vi "Autonomous Independent.vi"() -> ()   [LabVIEW 2016]
doc: "This VI is called when autonomous begins, and will automatically be terminated when autonomous ends. You can carry out timed or sensor driven robot movement independently without needing to return to the caller."
uses:
  Robot Global Data.vi
  <vilib>/addons/control/pid/pid.llb/PID (DBL).vi
  navX Library v2/navX Library v2.lvlib
  <vilib>/addons/control/pid/NI_PID_pid.lvlib
  <vilib>/Rock Robotics/Network Tables/NT Read String.vi
panel:
  out "x+y":dbl
  out "x-y":dbl
  out "Numeric 2":i32
  out "elapsed time":i32
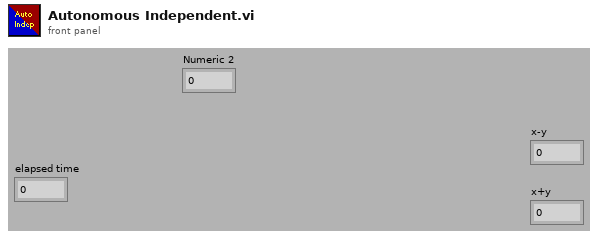
[diagram p1: front panel]
types:
  T1 = typedef "navX Library v2.lvlib/Z900_navX_DeviceTypeDef.ctl" = cluster{"Interface":cluster{"Protocol":T2, "Update Rate (4Hz-100Hz)":u8, "navX Open TypeDef":variant}, "Notify Packet":refnum<notifier>, "Loop VI Refnum":refnum<vi>, "Ready to Close Occurrence Refnum":refnum<k4>}
  T2 = typedef "navX Library v2.lvlib/Z900_navX_ProtocolTypeDef.ctl" = enum16{"SERIAL", "I2C", "SPI"}
  T3 = typedef "WPI_EncoderDevRef.ctl" = cluster{"DevStatus":errorcluster, "EncoderIndex":T4, "CounterIndex":T5, "DistancePerCount":dbl, "Decoding Type":T6}
  T4 = typedef "FPGA_EncoderIdx.ctl" = enum8{"Enc 0", "Enc 1", "Enc 2", "Enc 3", "Enc 4", "Enc 5", "Enc 6", "Enc 7", "Invalid"}
  T5 = typedef "FPGA_CounterCtrSystemIndex.ctl" = enum8{"Ctr 0", "Ctr 1", "Ctr 2", "Ctr 3", "Ctr 4", "Ctr 5", "Ctr 6", "Ctr 7", "Invalid"}
  T6 = typedef "WPI_EncoderType.ctl" = enum16{"1x", "2x", "4x"}
  T7 = cluster{"proportional gain (Kc)":dbl, "integral time (Ti, min)":dbl, "derivative time (Td, min)":dbl}
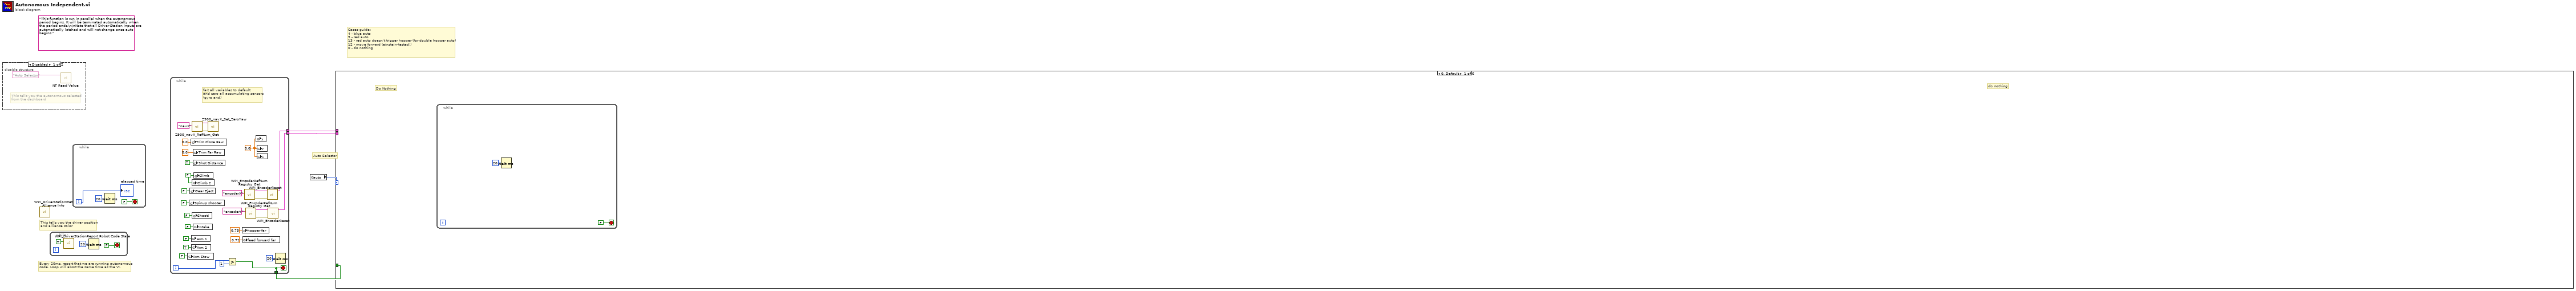
[diagram p0: block diagram]
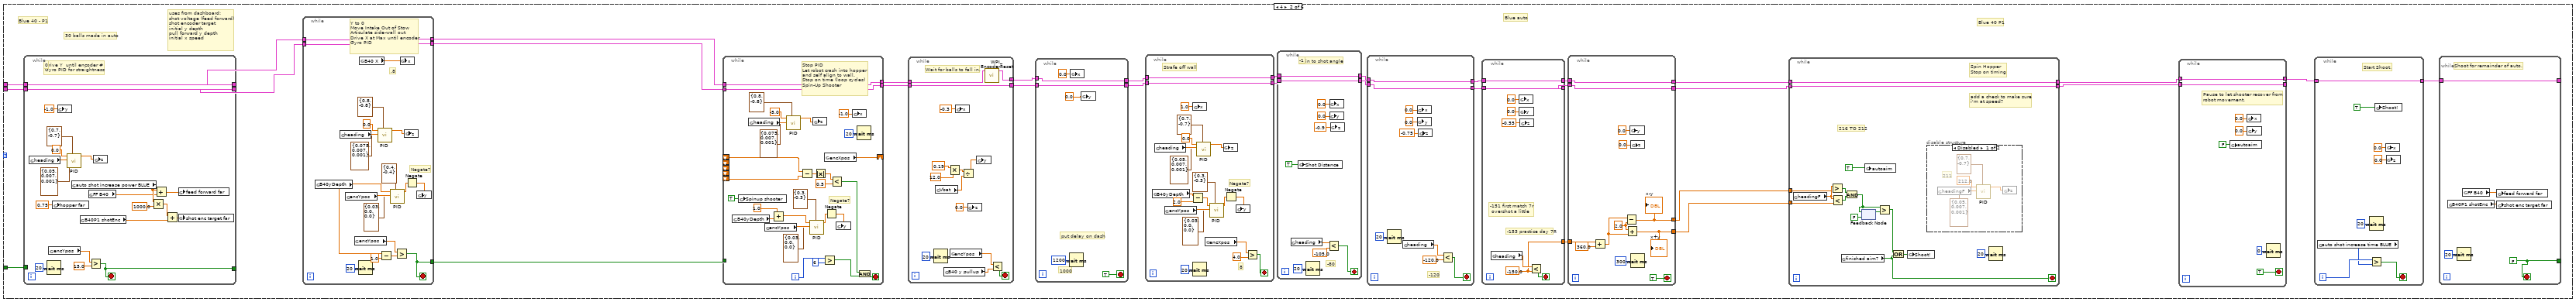
[diagram p2: hidden frame]
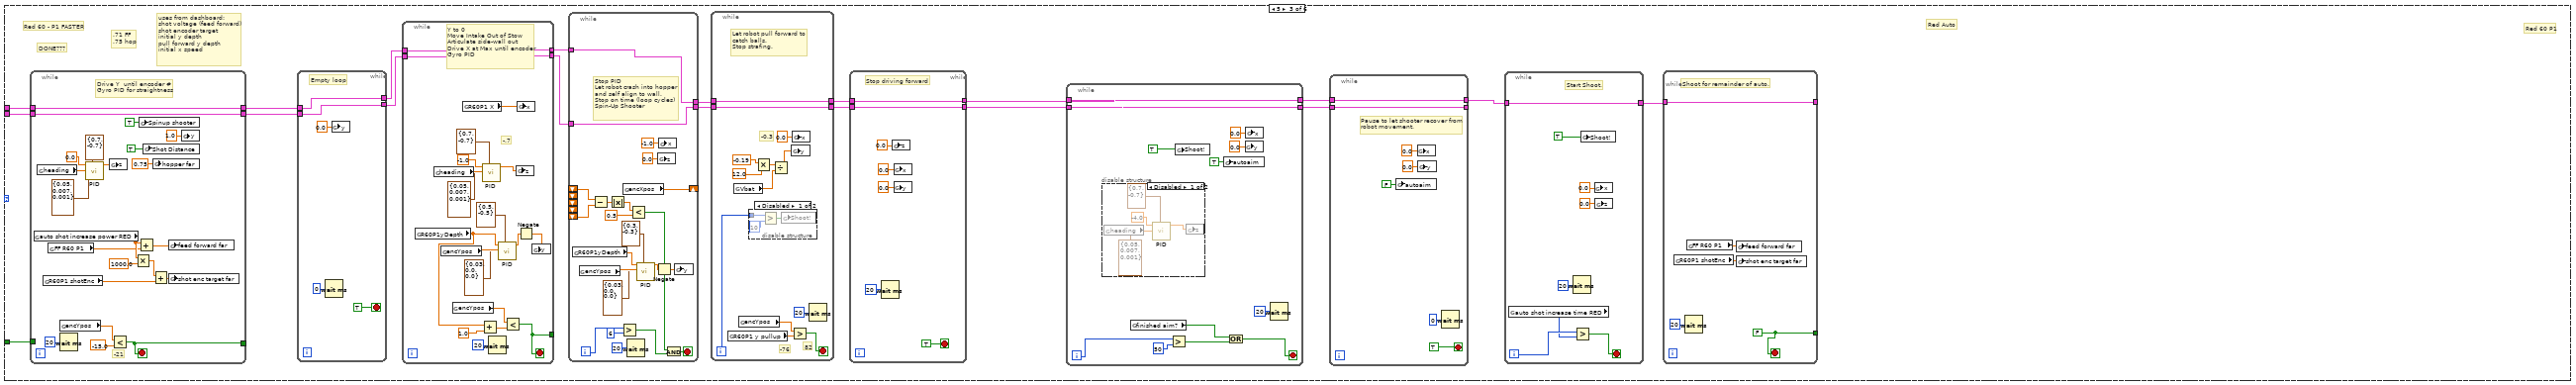
[diagram p4: hidden frame]
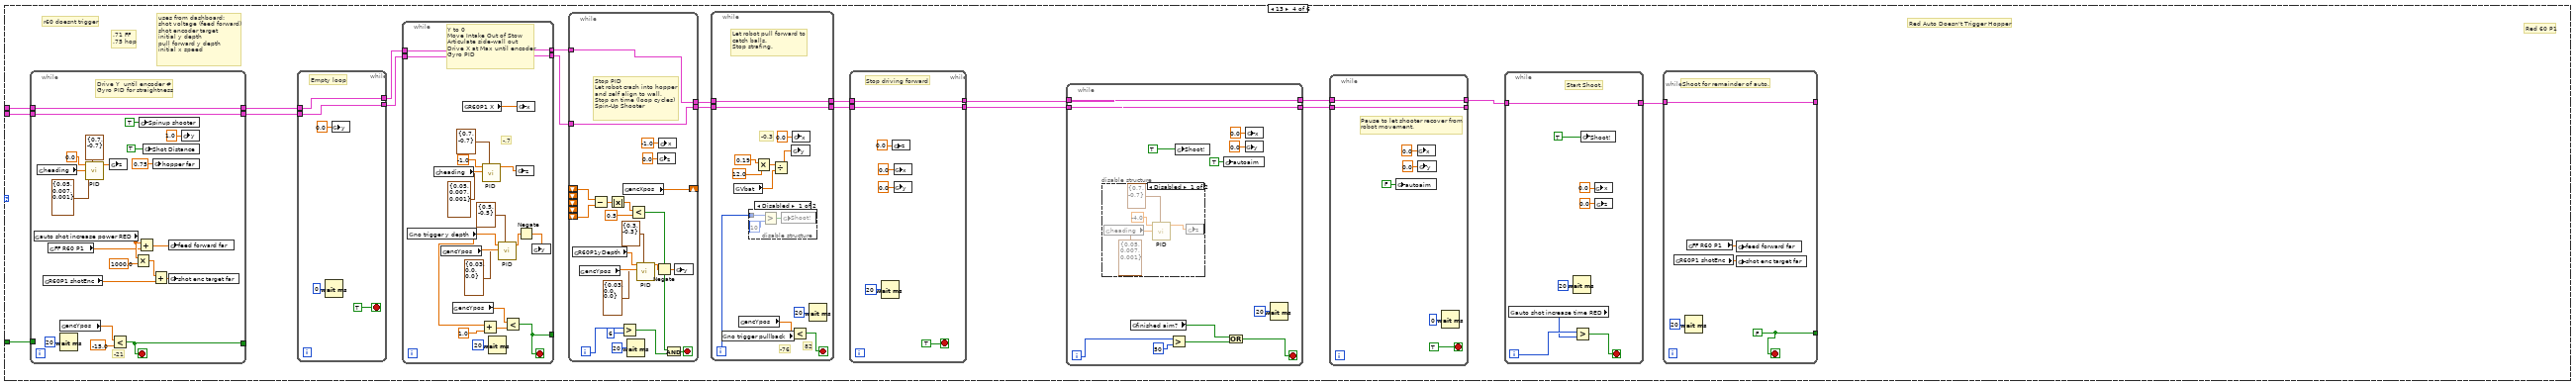
[diagram p7: hidden frame]
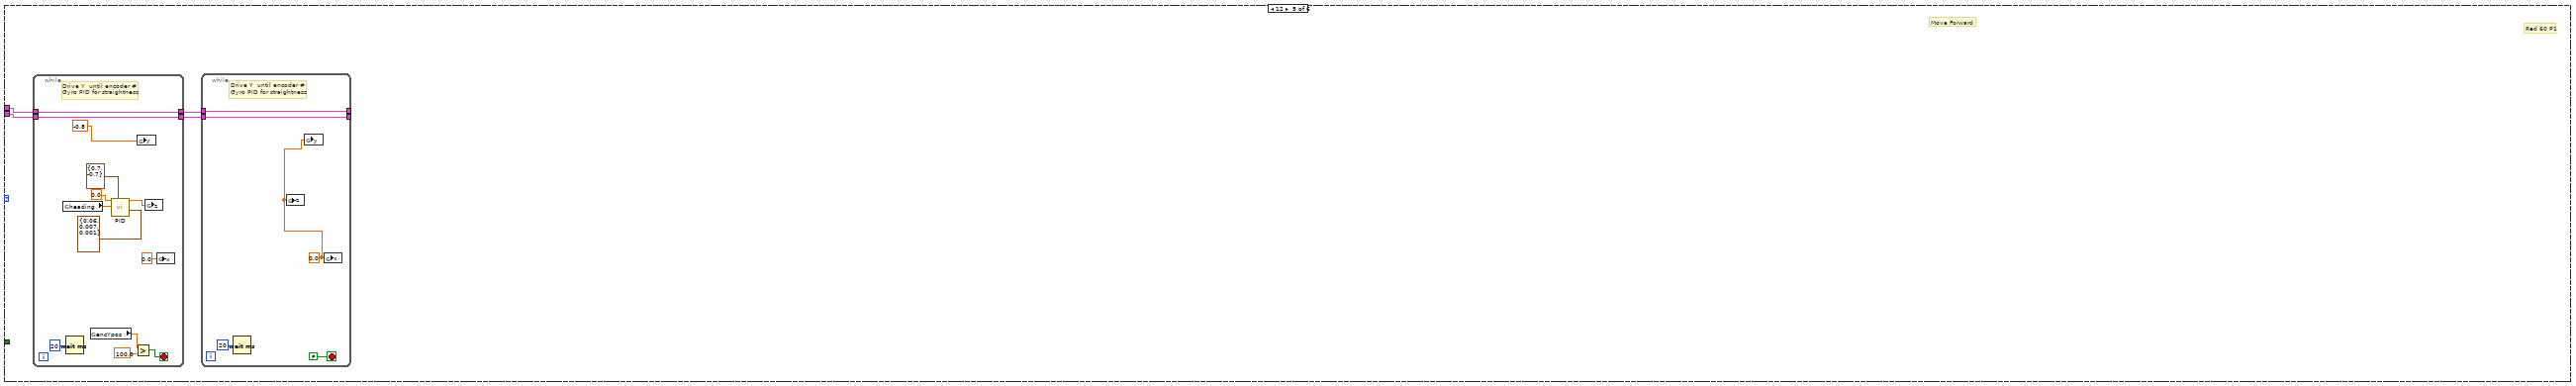
[diagram p10: hidden frame]
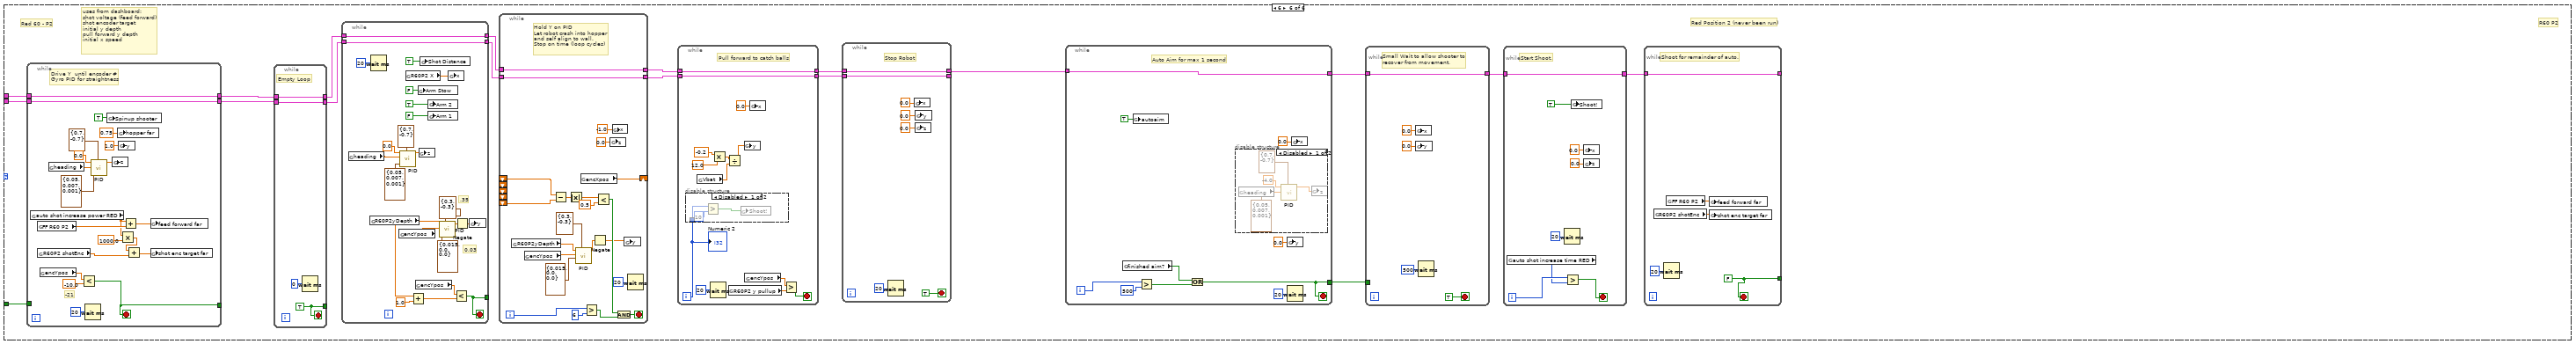
[diagram p11: hidden frame]
diagram:
  (unwired) "This function is run in parallel when the autonomous period begins. It will be terminated automatically when the period ends.\n\nNote that all Driver Station inputs are automatically latched and will not change once auto begins."
  # "Cases guide:\n4 - blue auto\n5 - red auto\n13 - red auto doesn't trigger hopper (for double hopper auto)\n12 - move forward (einstein-tested!)\n0 - do nothing"
  # "Auto Selector"
  # "Every 20ms, report that we are running autonomous\ncode. Loop will abort the same time as the VI."
  # "This tells you the driver position\nand alliance color"
  n1 = disable-structure shown="Disabled" {
    frame Disabled {
      # "This tells you the autonomous selected\nfrom the dashboard"
      n2 = call-poly <vilib>:"NT Read Value.vi"("Name"="Auto Selector") -> ()  [unwired: 9 in, 2 out]
    }
    frame Enabled {
    }
  }
  n3 = call <vilib>:"WPI_DriverStationGet Alliance Info.vi"() -> ()  [unwired: 12 out]
  n4 = while {
    stop <- FALSE stop-if-true
    n5 = call <vilib>:"WPI_DriverStationReport Robot Code State.vi"("Autonomous"=TRUE) -> ()  [unwired: 10 in, 1 out]
    n6 = Wait (ms)(milliseconds to wait=u32 20) -> ()  [unwired: 1 out]
  }
  n7 = while {
    i -> [w9]
    stop <- FALSE stop-if-true
    n8 = Wait (ms)(milliseconds to wait=u32 20) -> ()  [unwired: 1 out]
    "elapsed time" <- w9
  }
  n9 = while {
    tunnel: [w18] -> w4
    tunnel: [w21] -> w2
    tunnel: [w12] -> w1
    i -> [w20]
    stop <- w18 stop-if-true
    w28 = 0.0 ("y")
    w36 = FALSE ("Climb")
    # "far"
    # "Set all variables to default\nand zero all accumulating sensors\n(gyro and)"
    n10 = global write "Robot Global Data.vi" "Arm Stow"(FALSE ("Arm Stow")) -> ()
    n11 = global write "Robot Global Data.vi" "Spinup shooter"(FALSE ("Spinup shooter")) -> ()
    n12 = global write "Robot Global Data.vi" "Gear Eject"(FALSE ("Gear Eject")) -> ()
    n13 = global write "Robot Global Data.vi" "Trim Close Raw"(0.0 ("Trim Close Raw")) -> ()
    n14 = global write "Robot Global Data.vi" "Arm 1"(FALSE ("Arm 1")) -> ()
    n15 = global write "Robot Global Data.vi" "Arm 2"(TRUE ("Arm 2")) -> ()
    n16 = call "Z900_navX_RefNum_Get.vi"("refnum name"="navX") -> ("error out"=w15:errorcluster, "navX Device"=w14:T1)  [unwired: 9 in]
    n17 = global write "Robot Global Data.vi" "Climb 2"(w36) -> ()
    n18 = global write "Robot Global Data.vi" "Shoot!"(FALSE ("Shoot!")) -> ()
    n19 = global write "Robot Global Data.vi" "Trim Far Raw"(0.0 ("Trim Close Raw")) -> ()
    n20 = global write "Robot Global Data.vi" "Shot Distance"(TRUE ("Shot Distance")) -> ()
    n21 = global write "Robot Global Data.vi" "Intake"(FALSE ("Intake")) -> ()
    n22 = global write "Robot Global Data.vi" "Climb"(w36) -> ()
    n23 = call "Z900_navX_Set_ZeroYaw.vi"("error in (no error)"=w15, "navX Device"=w14) -> ()  [unwired: 8 in, 2 out]
    n24 = Greater?(x=w20, y=1) -> (0:w18:bool)
    n25 = global write "Robot Global Data.vi" "hopper far"(0.75 ("hopper far")) -> ()
    n26 = global write "Robot Global Data.vi" "feed forward far"(0.71 ("feed forward far")) -> ()
    n27 = call <vilib>:"WPI_EncoderRefNum Registry Get.vi"("refnum name"="encoderX") -> ("error out"=w26:errorcluster, "EncoderDevRef"=w27:T3)  [unwired: 9 in]
    n28 = call <vilib>:"WPI_EncoderRefNum Registry Get.vi"("refnum name"="encoderY") -> ("error out"=w24:errorcluster, "EncoderDevRef"=w25:T3)  [unwired: 9 in]
    n29 = global write "Robot Global Data.vi" "x"(w28) -> ()
    n30 = global write "Robot Global Data.vi" "y"(w28) -> ()
    n31 = global write "Robot Global Data.vi" "z"(w28) -> ()
    n32 = call <vilib>:"WPI_EncoderReset.vi"("error in (no error)"=w26, "EncoderDevRef"=w27) -> ("EncoderDevRef"=w21:T3)  [unwired: 8 in, 1 out]
    n33 = call <vilib>:"WPI_EncoderReset.vi"("error in (no error)"=w24, "EncoderDevRef"=w25) -> ("EncoderDevRef"=w12:T3)  [unwired: 8 in, 1 out]
    n34 = Wait (ms)(milliseconds to wait=u32 20) -> ()  [unwired: 1 out]
  }
  n35 = global read "Robot Global Data.vi" "auto"() -> (w3:i32)
  n36 = case shown="0, Default" w3 {
    tunnel: w4 -> [_ w73 w279 w426 _ w594]
    tunnel: w2 -> [_ w72 w278 w425 w558 w593]
    tunnel: w1 -> [_ w71 w277 w424 w557 w592]
    frame 0, Default {
      # "Do Nothing"
      # "do nothing"
      n37 = while {
        stop <- FALSE stop-if-true
        n38 = Wait (ms)(milliseconds to wait=u32 20) -> ()  [unwired: 1 out]
      }
    }
    frame 4 {
      # "Blue auto"
      # "uses from dashboard:\nshot voltage (feed forward)\nshot encoder target\ninitial y depth\npull forward y depth\ninitial x speed"
      # "30 balls made in auto"
      # "Blue 40 P1"
      # "Blue 40 - P1"
      n39 = while {
        tunnel: w73 -> [_]
        tunnel: [w252] -> _
        tunnel: [w251] -> w67
        tunnel: w72 -> [w251]
        tunnel: [w250] -> w66
        tunnel: w71 -> [w250]
        stop <- w252 stop-if-true
        # "0"
        # "Drive Y  until encoder #\nGyro PID for straightness"
        n40 = global read "Robot Global Data.vi" "heading"() -> (w258:dbl)
        n41 = Wait (ms)(milliseconds to wait=u32 20) -> ()  [unwired: 1 out]
        n42 = global read "Robot Global Data.vi" "encYpos"() -> (w255:dbl)
        n43 = global write "Robot Global Data.vi" "hopper far"(0.75 ("hopper far")) -> ()
        n44 = global write "Robot Global Data.vi" "y"(-1.0 ("y")) -> ()
        n45 = call-poly <vilib>:"PID.vi"("output range"=cluster{"output high":dbl, "output low":dbl} {"output high"=0.7, "output low"=-0.7}, "PID gains"=T7 {"proportional gain (Kc)"=0.05, "integral time (Ti, min)"=0.007, "derivative time (Td, min)"=0.001}, "process variable"=w258, "setpoint"=0.0) -> ("output"=w256:dbl)  [unwired: 6 in, 1 out]
        n46 = global read "Robot Global Data.vi" "auto shot increase power BLUE"() -> (w246:dbl)
        n47 = global read "Robot Global Data.vi" "B40P1 shotEnc"() -> (w243:dbl)
        n48 = global read "Robot Global Data.vi" "FF B40"() -> (w242:dbl)
        n49 = Greater?(x=w255, y=15.0) -> (0:w252:bool)
        n50 = global write "Robot Global Data.vi" "z"(w256) -> ()
        n51 = Multiply(x=w246, y=1000.0) -> (x*y=w244:dbl)
        n52 = Add(x=w246, y=w242) -> (x+y=w247:dbl)
        n53 = Add(x=w244, y=w243) -> (x+y=w241:dbl)
        n54 = global write "Robot Global Data.vi" "feed forward far"(w247) -> ()
        n55 = global write "Robot Global Data.vi" "shot enc target far"(w241) -> ()
      }
      n56 = while {
        tunnel: [w240] -> w70
        tunnel: w67 -> [w240]
        tunnel: w66 -> [w239]
        tunnel: [w239] -> w69
        tunnel: [w232] -> w68
        stop <- w232 stop-if-true
        # ".8"
        # "Negate?"
        # "Y to 0\nMove Intake Out of Stow\nArticulate side-wall out\nDrive X at Max until encoder\nGyro PID"
        n57 = global read "Robot Global Data.vi" "B40yDepth"() -> (w224:dbl)
        n58 = global read "Robot Global Data.vi" "heading"() -> (w236:dbl)
        n59 = global read "Robot Global Data.vi" "encYpos"() -> (w229:dbl)
        n60 = global read "Robot Global Data.vi" "encYpos"() -> (w233:dbl)
        n61 = Wait (ms)(milliseconds to wait=u32 20) -> ()  [unwired: 1 out]
        n62 = global read "Robot Global Data.vi" "B40 X"() -> (w222:dbl)
        n63 = call-poly <vilib>:"PID.vi"("output range"=cluster{"output high":dbl, "output low":dbl} {"output high"=0.8, "output low"=-0.8}, "PID gains"=T7 {"proportional gain (Kc)"=0.075, "integral time (Ti, min)"=0.007, "derivative time (Td, min)"=0.001}, "process variable"=w236, "setpoint"=0.0) -> ("output"=w234:dbl)  [unwired: 6 in, 1 out]
        n64 = Subtract(x=w224, y=1.0) -> (x-y=w225:dbl)
        n65 = call-poly <vilib>:"PID.vi"("output range"=cluster{"output high":dbl, "output low":dbl} {"output high"=0.4, "output low"=-0.4}, "PID gains"=T7 {"proportional gain (Kc)"=0.03, "integral time (Ti, min)"=0.0, "derivative time (Td, min)"=0.0}, "process variable"=w229, "setpoint"=w224) -> ("output"=w227:dbl)  [unwired: 6 in, 1 out]
        n66 = Greater?(x=w233, y=w225) -> (0:w232:bool)
        n67 = global write "Robot Global Data.vi" "x"(w222) -> ()
        n68 = global write "Robot Global Data.vi" "z"(w234) -> ()
        n69 = Negate(x=w227) -> (-x=w226:dbl)
        n70 = global write "Robot Global Data.vi" "y"(w226) -> ()
      }
      n71 = while {
        tunnel: [w221] -> w65
        tunnel: w70 -> [w221]
        tunnel: w69 -> [w220]
        tunnel: [w220] -> w64
        tunnel: w68 -> [_]
        shift-right: [w217] -> _
        shift-left: _ -> [w216]
        shift-left: _ -> [_]
        shift-left: _ -> [_]
        shift-left: _ -> [_]
        shift-left: _ -> [w212]
        i -> [w208]
        stop <- w211 stop-if-true
        # "Negate?"
        # "Stop PID\nLet robot crash into hopper\nand self align to wall.\nStop on time (loop cycles)\nSpin-Up Shooter"
        n72 = global read "Robot Global Data.vi" "B40yDepth"() -> (w195:dbl)
        n73 = global write "Robot Global Data.vi" "Spinup shooter"(TRUE ("Spinup shooter")) -> ()
        n74 = global read "Robot Global Data.vi" "heading"() -> (w200:dbl)
        n75 = global read "Robot Global Data.vi" "encYpos"() -> (w205:dbl)
        n76 = Add(x=1.0, y=w195) -> (x+y=w193:dbl)
        n77 = call-poly <vilib>:"PID.vi"("output range"=cluster{"output high":dbl, "output low":dbl} {"output high"=0.8, "output low"=-0.8}, "PID gains"=T7 {"proportional gain (Kc)"=0.075, "integral time (Ti, min)"=0.007, "derivative time (Td, min)"=0.001}, "process variable"=w200, "setpoint"=-5.0) -> ("output"=w198:dbl)  [unwired: 6 in, 1 out]
        n78 = Subtract(x=w216, y=w212) -> (x-y=w215:dbl)
        n79 = call-poly <vilib>:"PID.vi"("output range"=cluster{"output high":dbl, "output low":dbl} {"output high"=0.3, "output low"=-0.3}, "PID gains"=T7 {"proportional gain (Kc)"=0.03, "integral time (Ti, min)"=0.0, "derivative time (Td, min)"=0.0}, "process variable"=w205, "setpoint"=w193) -> ("output"=w203:dbl)  [unwired: 6 in, 1 out]
        n80 = global write "Robot Global Data.vi" "z"(w198) -> ()
        n81 = Absolute Value(x=w215) -> (abs(x)=w214:dbl)
        n82 = Greater?(x=w208, y=6) -> (0:w210:bool)
        n83 = global read "Robot Global Data.vi" "encXpos"() -> (w217:dbl)
        n84 = Negate(x=w203) -> (-x=w202:dbl)
        n85 = Less?(x=w214, y=0.5) -> (x < y?=w209:bool)
        n86 = global write "Robot Global Data.vi" "y"(w202) -> ()
        n87 = global write "Robot Global Data.vi" "x"(-1.0 ("x")) -> ()
        n88 = Wait (ms)(milliseconds to wait=u32 20) -> ()  [unwired: 1 out]
        n89 = And(x=w209, y=w210) -> (x .and. y?=w211:bool)
      }
      n90 = while {
        tunnel: w65 -> [w169]
        tunnel: w64 -> [w170]
        tunnel: [w168] -> w63
        tunnel: [w170] -> w61
        stop <- w161 stop-if-true
        # "Wait for balls to fall in."
        n91 = Wait (ms)(milliseconds to wait=u32 20) -> ()  [unwired: 1 out]
        n92 = global read "Robot Global Data.vi" "Vbat"() -> (w164:dbl)
        n93 = global read "Robot Global Data.vi" "B40 y pullup"() -> (w159:dbl)
        n94 = Multiply(x=0.19 ("y"), y=12.0) -> (x*y=w166:dbl)
        n95 = global read "Robot Global Data.vi" "encYpos"() -> (w162:dbl)
        n96 = global write "Robot Global Data.vi" "x"(-0.3 ("x")) -> ()
        n97 = Divide(x=w166, y=w164) -> (x/y=w163:dbl)
        n98 = global write "Robot Global Data.vi" "z"(0.0 ("y")) -> ()
        n99 = global write "Robot Global Data.vi" "y"(w163) -> ()
        n100 = call <vilib>:"WPI_EncoderReset.vi"("EncoderDevRef"=w169) -> ("EncoderDevRef"=w168:T3)  [unwired: 9 in, 1 out]
        n101 = Less?(x=w162, y=w159) -> (x < y?=w161:bool)
      }
      n102 = while {
        tunnel: w63 -> [w135]
        tunnel: [w135] -> w62
        tunnel: w61 -> [w134]
        tunnel: [w134] -> w60
        stop <- TRUE stop-if-true
        # "put delay on dash"
        # "1000"
        n103 = Wait (ms)(milliseconds to wait=u32 1200) -> ()  [unwired: 1 out]
        n104 = global write "Robot Global Data.vi" "x"(0.0 ("x")) -> ()
        n105 = global write "Robot Global Data.vi" "y"(0.0 ("x")) -> ()
      }
      n106 = while {
        tunnel: w62 -> [w156]
        tunnel: w60 -> [w155]
        tunnel: [w156] -> w54
        tunnel: [w155] -> w55
        stop <- w142 stop-if-true
        # "8"
        # "Negate?"
        # "Strafe off wall"
        n107 = global read "Robot Global Data.vi" "B40yDepth"() -> (w141:dbl)
        n108 = global read "Robot Global Data.vi" "heading"() -> (w152:dbl)
        n109 = global read "Robot Global Data.vi" "encYpos"() -> (w148:dbl)
        n110 = Subtract(x=w141, y=2.0) -> (x-y=w140:dbl)
        n111 = global write "Robot Global Data.vi" "x"(1.0 ("x")) -> ()
        n112 = Wait (ms)(milliseconds to wait=u32 20) -> ()  [unwired: 1 out]
        n113 = call-poly <vilib>:"PID.vi"("output range"=cluster{"output high":dbl, "output low":dbl} {"output high"=0.7, "output low"=-0.7}, "PID gains"=T7 {"proportional gain (Kc)"=0.05, "integral time (Ti, min)"=0.007, "derivative time (Td, min)"=0.001}, "process variable"=w152, "setpoint"=0.0) -> ("output"=w150:dbl)  [unwired: 6 in, 1 out]
        n114 = global read "Robot Global Data.vi" "encXpos"() -> (w144:dbl)
        n115 = call-poly <vilib>:"PID.vi"("output range"=cluster{"output high":dbl, "output low":dbl} {"output high"=0.3, "output low"=-0.3}, "PID gains"=T7 {"proportional gain (Kc)"=0.03, "integral time (Ti, min)"=0.0, "derivative time (Td, min)"=0.0}, "process variable"=w148, "setpoint"=w140) -> ("output"=w146:dbl)  [unwired: 6 in, 1 out]
        n116 = global write "Robot Global Data.vi" "z"(w150) -> ()
        n117 = Negate(x=w146) -> (-x=w145:dbl)
        n118 = global write "Robot Global Data.vi" "y"(w145) -> ()
        n119 = Greater?(x=w144, y=4.0) -> (0:w142:bool)
      }
      n120 = while {
        tunnel: [w111] -> w57
        tunnel: w54 -> [w111]
        tunnel: [w110] -> w56
        tunnel: w55 -> [w110]
        stop <- w105 stop-if-true
        # "-1"
        # "-80"
        # "Spin to shot angle"
        n121 = global read "Robot Global Data.vi" "heading"() -> (w106:dbl)
        n122 = global write "Robot Global Data.vi" "Shot Distance"(TRUE ("Spinup shooter")) -> ()
        n123 = Wait (ms)(milliseconds to wait=u32 20) -> ()  [unwired: 1 out]
        n124 = Less?(x=w106, y=-105.0) -> (x < y?=w105:bool)
        n125 = global write "Robot Global Data.vi" "x"(0.0 ("x")) -> ()
        n126 = global write "Robot Global Data.vi" "y"(0.0 ("x")) -> ()
        n127 = global write "Robot Global Data.vi" "z"(-0.9 ("z")) -> ()
      }
      n128 = while {
        tunnel: w57 -> [w131]
        tunnel: [w131] -> w53
        tunnel: w56 -> [w130]
        tunnel: [w130] -> w51
        stop <- w129 stop-if-true
        # "-120"
        n129 = Wait (ms)(milliseconds to wait=u32 20) -> ()  [unwired: 1 out]
        n130 = global read "Robot Global Data.vi" "heading"() -> (w128:dbl)
        n131 = global write "Robot Global Data.vi" "x"(0.0 ("x")) -> ()
        n132 = global write "Robot Global Data.vi" "y"(0.0 ("x")) -> ()
        n133 = global write "Robot Global Data.vi" "z"(-0.75 ("z")) -> ()
        n134 = Less?(x=w128, y=-120.0) -> (x < y?=w129:bool)
      }
      n135 = while {
        tunnel: w53 -> [w96]
        tunnel: [w96] -> w52
        tunnel: w51 -> [w95]
        tunnel: [w95] -> w50
        tunnel: [w94] -> w49
        stop <- w97 stop-if-true
        w94 = -150.0 ("y")
        # "-151 first match 7r\n overshot a little"
        # "-153 practice day 7R"
        n136 = global read "Robot Global Data.vi" "heading"() -> (w98:dbl)
        n137 = global write "Robot Global Data.vi" "x"(0.0 ("x")) -> ()
        n138 = global write "Robot Global Data.vi" "y"(0.0 ("x")) -> ()
        n139 = global write "Robot Global Data.vi" "z"(-0.55 ("z")) -> ()
        n140 = Less?(x=w98, y=w94) -> (x < y?=w97:bool)
      }
      n141 = while {
        tunnel: w52 -> [w121]
        tunnel: [w121] -> w59
        tunnel: w50 -> [w120]
        tunnel: [w120] -> w58
        tunnel: w49 -> [w117]
        tunnel: [w115] -> w48
        tunnel: [w112] -> w47
        stop <- TRUE stop-if-true
        w114 = 2.0 ("y")
        n142 = Add(x=w117, y=360.0) -> (x+y=w113:dbl)
        n143 = Subtract(x=w113, y=w114) -> (x-y=w115:dbl)
        "x-y" <- w115
        n144 = Add(x=w114, y=w113) -> (x+y=w112:dbl)
        "x+y" <- w112
        n145 = global write "Robot Global Data.vi" "y"(0.0 ("x")) -> ()
        n146 = Wait (ms)(milliseconds to wait=u32 300) -> ()  [unwired: 1 out]
        n147 = global write "Robot Global Data.vi" "z"(0.0 ("z")) -> ()
      }
      n148 = while {
        tunnel: [w187] -> w44
        tunnel: w59 -> [w187]
        tunnel: w58 -> [w186]
        tunnel: [w186] -> w43
        tunnel: w48 -> [w175]
        tunnel: w47 -> [w174]
        stop <- w173 stop-if-true
        # "216 TO 212"
        # "add a check to make sure\ni'm at speed?"
        # "Spin Hopper\nStop on timing"
        n149 = global read "Robot Global Data.vi" "headingF"() -> (w181:dbl)
        n150 = Greater?(x=w181, y=w175) -> (0:w183:bool)
        n151 = Less?(x=w181, y=w174) -> (x < y?=w182:bool)
        n152 = global read "Robot Global Data.vi" "finished aim?"() -> (w173:bool)
        n153 = And(x=w183, y=w182) -> (x .and. y?=w178:bool)
        n154 = feedback #1(FALSE) -> (w179:bool)
        n155 = feedback-in #1(w178) -> ()
        n156 = global write "Robot Global Data.vi" "autoaim"(TRUE ("Spinup shooter")) -> ()
        n157 = Greater?(x=w178, y=w179) -> (0:w177:bool)
        n158 = Or(x=w177, y=w173) -> (x .or. y?=w180:bool)
        n159 = global write "Robot Global Data.vi" "Shoot!"(w180) -> ()
        n160 = disable-structure shown="Disabled" {
          frame Disabled {
            # "211"
            n161 = global read "Robot Global Data.vi" "headingF"() -> (w190:dbl)
            n162 = call-poly <vilib>:"PID.vi"("output range"=cluster{"output high":dbl, "output low":dbl} {"output high"=0.7, "output low"=-0.7}, "PID gains"=T7 {"proportional gain (Kc)"=0.05, "integral time (Ti, min)"=0.007, "derivative time (Td, min)"=0.001}, "process variable"=w190, "setpoint"=212.0) -> ("output"=w188:dbl)  [unwired: 6 in, 1 out]
            n163 = global write "Robot Global Data.vi" "z"(w188) -> ()
          }
          frame Enabled {
          }
        }
        n164 = Wait (ms)(milliseconds to wait=u32 20) -> ()  [unwired: 1 out]
      }
      n165 = while {
        tunnel: [w93] -> w45
        tunnel: w44 -> [w93]
        tunnel: [w92] -> _
        tunnel: w43 -> [w92]
        stop <- TRUE stop-if-true
        # "Pause to let shooter recover from\nrobot movement."
        n166 = global write "Robot Global Data.vi" "autoaim"(FALSE ("autoaim")) -> ()
        n167 = global write "Robot Global Data.vi" "x"(0.0 ("x")) -> ()
        n168 = global write "Robot Global Data.vi" "y"(0.0 ("y")) -> ()
        n169 = Wait (ms)(milliseconds to wait=u32 0) -> ()  [unwired: 1 out]
      }
      n170 = while {
        tunnel: w45 -> [w86]
        tunnel: [w86] -> w46
        i -> [w81]
        stop <- w80 stop-if-true
        # "Start Shoot."
        n171 = global read "Robot Global Data.vi" "auto shot increase time BLUE"() -> (w79:i32)
        n172 = Wait (ms)(milliseconds to wait=u32 20) -> ()  [unwired: 1 out]
        n173 = Greater?(x=w81, y=w79) -> (0:w80:bool)
        n174 = global write "Robot Global Data.vi" "Shoot!"(TRUE ("Spinup shooter")) -> ()
        n175 = global write "Robot Global Data.vi" "x"(0.0 ("x")) -> ()
        n176 = global write "Robot Global Data.vi" "z"(0.0 ("z")) -> ()
      }
      n177 = while {
        tunnel: w46 -> [w78]
        tunnel: [w78] -> _
        tunnel: [w76] -> _
        stop <- w76 stop-if-true
        w76 = FALSE
        # "Shoot for remainder of auto."
        n178 = global read "Robot Global Data.vi" "B40P1 shotEnc"() -> (w74:dbl)
        n179 = Wait (ms)(milliseconds to wait=u32 20) -> ()  [unwired: 1 out]
        n180 = global read "Robot Global Data.vi" "FF B40"() -> (w75:dbl)
        n181 = global write "Robot Global Data.vi" "feed forward far"(w75) -> ()
        n182 = global write "Robot Global Data.vi" "shot enc target far"(w74) -> ()
      }
    }
    frame 5 {
      # "Red Auto"
      # "uses from dashboard:\nshot voltage (feed forward)\nshot encoder target\ninitial y depth\npull forward y depth\ninitial x speed"
      # ".71 FF\n.75 hop"
      # "DONE???"
      # "Red 60 P1"
      # "Red 60 - P1 FASTER"
      n183 = while {
        tunnel: w279 -> [_]
        tunnel: [w399] -> _
        tunnel: [w398] -> w276
        tunnel: w278 -> [w398]
        tunnel: [w397] -> w274
        tunnel: w277 -> [w397]
        stop <- w399 stop-if-true
        # "-21"
        # "Drive Y  until encoder #\nGyro PID for straightness"
        n184 = global read "Robot Global Data.vi" "auto shot increase power RED"() -> (w391:dbl)
        n185 = global read "Robot Global Data.vi" "heading"() -> (w405:dbl)
        n186 = global read "Robot Global Data.vi" "R60P1 shotEnc"() -> (w388:dbl)
        n187 = global read "Robot Global Data.vi" "FF R60 P1"() -> (w387:dbl)
        n188 = global read "Robot Global Data.vi" "encYpos"() -> (w402:dbl)
        n189 = Wait (ms)(milliseconds to wait=u32 20) -> ()  [unwired: 1 out]
        n190 = call-poly <vilib>:"PID.vi"("output range"=cluster{"output high":dbl, "output low":dbl} {"output high"=0.7, "output low"=-0.7}, "PID gains"=T7 {"proportional gain (Kc)"=0.05, "integral time (Ti, min)"=0.007, "derivative time (Td, min)"=0.001}, "process variable"=w405, "setpoint"=0.0) -> ("output"=w403:dbl)  [unwired: 6 in, 1 out]
        n191 = global write "Robot Global Data.vi" "z"(w403) -> ()
        n192 = Less?(x=w402, y=-15.0) -> (x < y?=w399:bool)
        n193 = Multiply(x=w391, y=1000.0) -> (x*y=w389:dbl)
        n194 = Add(x=w391, y=w387) -> (x+y=w392:dbl)
        n195 = global write "Robot Global Data.vi" "Spinup shooter"(TRUE ("Spinup shooter")) -> ()
        n196 = global write "Robot Global Data.vi" "Shot Distance"(TRUE ("Spinup shooter")) -> ()
        n197 = Add(x=w389, y=w388) -> (x+y=w386:dbl)
        n198 = global write "Robot Global Data.vi" "hopper far"(0.75 ("hopper far")) -> ()
        n199 = global write "Robot Global Data.vi" "feed forward far"(w392) -> ()
        n200 = global write "Robot Global Data.vi" "shot enc target far"(w386) -> ()
        n201 = global write "Robot Global Data.vi" "y"(1.0 ("y")) -> ()
      }
      n202 = while {
        tunnel: [w328] -> w275
        tunnel: w276 -> [w328]
        tunnel: w274 -> [w325]
        tunnel: [w325] -> w273
        stop <- TRUE stop-if-true
        # "Empty loop"
        n203 = Wait (ms)(milliseconds to wait=u32 0) -> ()  [unwired: 1 out]
        n204 = global write "Robot Global Data.vi" "y"(0.0 ("y")) -> ()
      }
      n205 = while {
        tunnel: [w385] -> w272
        tunnel: w275 -> [w385]
        tunnel: w273 -> [w384]
        tunnel: [w384] -> w271
        tunnel: [w377] -> _
        stop <- w377 stop-if-true
        # "-.7"
        # "Y to 0\nMove Intake Out of Stow\nArticulate side-wall out\nDrive X at Max until encoder\nGyro PID"
        n206 = global read "Robot Global Data.vi" "R60P1yDepth"() -> (w367:dbl)
        n207 = global read "Robot Global Data.vi" "heading"() -> (w381:dbl)
        n208 = global read "Robot Global Data.vi" "encYpos"() -> (w374:dbl)
        n209 = global read "Robot Global Data.vi" "encYpos"() -> (w378:dbl)
        n210 = global read "Robot Global Data.vi" "R60P1 X"() -> (w370:dbl)
        n211 = Add(x=w367, y=1.0) -> (x+y=w369:dbl)
        n212 = call-poly <vilib>:"PID.vi"("output range"=cluster{"output high":dbl, "output low":dbl} {"output high"=0.7, "output low"=-0.7}, "PID gains"=T7 {"proportional gain (Kc)"=0.05, "integral time (Ti, min)"=0.007, "derivative time (Td, min)"=0.001}, "process variable"=w381, "setpoint"=-1.0) -> ("output"=w379:dbl)  [unwired: 6 in, 1 out]
        n213 = Wait (ms)(milliseconds to wait=u32 20) -> ()  [unwired: 1 out]
        n214 = call-poly <vilib>:"PID.vi"("output range"=cluster{"output high":dbl, "output low":dbl} {"output high"=0.5, "output low"=-0.5}, "PID gains"=T7 {"proportional gain (Kc)"=0.03, "integral time (Ti, min)"=0.0, "derivative time (Td, min)"=0.0}, "process variable"=w374, "setpoint"=w367) -> ("output"=w372:dbl)  [unwired: 6 in, 1 out]
        n215 = Less?(x=w378, y=w369) -> (x < y?=w377:bool)
        n216 = global write "Robot Global Data.vi" "z"(w379) -> ()
        n217 = global write "Robot Global Data.vi" "x"(w370) -> ()
        n218 = Negate(x=w372) -> (-x=w371:dbl)
        n219 = global write "Robot Global Data.vi" "y"(w371) -> ()
      }
      n220 = while {
        tunnel: [w352] -> w270
        tunnel: [w351] -> w269
        shift-right: [w363] -> _
        shift-left: _ -> [w362]
        shift-left: _ -> [_]
        shift-left: _ -> [_]
        shift-left: _ -> [_]
        shift-left: _ -> [w358]
        tunnel: w272 -> [w352]
        tunnel: w271 -> [w351]
        i -> [w354]
        stop <- w357 stop-if-true
        # "Stop PID\nLet robot crash into hopper\nand self align to wall.\nStop on time (loop cycles)\nSpin-Up Shooter"
        n221 = global read "Robot Global Data.vi" "R60P1yDepth"() -> (w345:dbl)
        n222 = global read "Robot Global Data.vi" "encYpos"() -> (w349:dbl)
        n223 = Subtract(x=w362, y=w358) -> (x-y=w361:dbl)
        n224 = Absolute Value(x=w361) -> (abs(x)=w360:dbl)
        n225 = Greater?(x=w354, y=6) -> (0:w356:bool)
        n226 = global read "Robot Global Data.vi" "encXpos"() -> (w363:dbl)
        n227 = Wait (ms)(milliseconds to wait=u32 20) -> ()  [unwired: 1 out]
        n228 = Less?(x=w360, y=0.5) -> (x < y?=w355:bool)
        n229 = call-poly <vilib>:"PID.vi"("output range"=cluster{"output high":dbl, "output low":dbl} {"output high"=0.3, "output low"=-0.3}, "PID gains"=T7 {"proportional gain (Kc)"=0.03, "integral time (Ti, min)"=0.0, "derivative time (Td, min)"=0.0}, "process variable"=w349, "setpoint"=w345) -> ("output"=w347:dbl)  [unwired: 6 in, 1 out]
        n230 = Negate(x=w347) -> (-x=w346:dbl)
        n231 = global write "Robot Global Data.vi" "z"(0.0 ("y")) -> ()
        n232 = global write "Robot Global Data.vi" "x"(-1.0 ("x")) -> ()
        n233 = And(x=w355, y=w356) -> (x .and. y?=w357:bool)
        n234 = global write "Robot Global Data.vi" "y"(w346) -> ()
      }
      n235 = while {
        tunnel: [w341] -> w267
        tunnel: w270 -> [w341]
        tunnel: [w340] -> w268
        tunnel: w269 -> [w340]
        i -> [w330]
        stop <- w336 stop-if-true
        # "Let robot pull forward to\ncatch balls.\nStop strafing."
        # "-0.3"
        # "82"
        # "-76"
        n236 = global read "Robot Global Data.vi" "R60P1 y pullup"() -> (w329:dbl)
        n237 = global read "Robot Global Data.vi" "Vbat"() -> (w332:dbl)
        n238 = global read "Robot Global Data.vi" "encYpos"() -> (w337:dbl)
        n239 = disable-structure shown="Disabled" {
          disable-tunnel: w330 -> [w343 _]
          frame Disabled {
            n240 = Greater?(x=w343, y=10) -> (0:w342:bool)
            n241 = global write "Robot Global Data.vi" "Shoot!"(w342) -> ()
          }
          frame Enabled {
          }
        }
        n242 = Multiply(x=-0.19 ("y"), y=12.0) -> (x*y=w334:dbl)
        n243 = Divide(x=w334, y=w332) -> (x/y=w331:dbl)
        n244 = Greater?(x=w337, y=w329) -> (0:w336:bool)
        n245 = global write "Robot Global Data.vi" "y"(w331) -> ()
        n246 = global write "Robot Global Data.vi" "x"(0.0 ("x")) -> ()
        n247 = Wait (ms)(milliseconds to wait=u32 20) -> ()  [unwired: 1 out]
      }
      n248 = while {
        tunnel: [w323] -> w266
        tunnel: w267 -> [w323]
        tunnel: w268 -> [w320]
        tunnel: [w320] -> w265
        stop <- TRUE stop-if-true
        # "Stop driving forward"
        n249 = Wait (ms)(milliseconds to wait=u32 20) -> ()  [unwired: 1 out]
        n250 = global write "Robot Global Data.vi" "z"(0.0 ("y")) -> ()
        n251 = global write "Robot Global Data.vi" "x"(0.0 ("y")) -> ()
        n252 = global write "Robot Global Data.vi" "y"(0.0 ("y")) -> ()
      }
      n253 = while {
        tunnel: [w310] -> w264
        tunnel: w266 -> [w310]
        tunnel: [w309] -> w263
        tunnel: w265 -> [w309]
        i -> [w302]
        stop <- w301 stop-if-true
        n254 = disable-structure shown="Disabled" {
          frame Disabled {
            n255 = global read "Robot Global Data.vi" "heading"() -> (w314:dbl)
            n256 = call-poly <vilib>:"PID.vi"("output range"=cluster{"output high":dbl, "output low":dbl} {"output high"=0.7, "output low"=-0.7}, "PID gains"=T7 {"proportional gain (Kc)"=0.05, "integral time (Ti, min)"=0.007, "derivative time (Td, min)"=0.001}, "process variable"=w314, "setpoint"=-4.0) -> ("output"=w312:dbl)  [unwired: 6 in, 1 out]
            n257 = global write "Robot Global Data.vi" "z"(w312) -> ()
          }
          frame Enabled {
          }
        }
        n258 = global read "Robot Global Data.vi" "finished aim?"() -> (w305:bool)
        n259 = Greater?(x=w302, y=50) -> (0:w304:bool)
        n260 = global write "Robot Global Data.vi" "Shoot!"(TRUE ("Spinup shooter")) -> ()
        n261 = global write "Robot Global Data.vi" "autoaim"(TRUE ("autoaim")) -> ()
        n262 = Or(x=w305, y=w304) -> (x .or. y?=w301:bool)
        n263 = global write "Robot Global Data.vi" "y"(0.0 ("y")) -> ()
        n264 = global write "Robot Global Data.vi" "x"(0.0 ("x")) -> ()
        n265 = Wait (ms)(milliseconds to wait=u32 20) -> ()  [unwired: 1 out]
      }
      n266 = while {
        tunnel: [w299] -> w261
        tunnel: w264 -> [w299]
        tunnel: [w298] -> _
        tunnel: w263 -> [w298]
        stop <- TRUE stop-if-true
        # "Pause to let shooter recover from\nrobot movement."
        n267 = global write "Robot Global Data.vi" "autoaim"(FALSE ("autoaim")) -> ()
        n268 = global write "Robot Global Data.vi" "x"(0.0 ("x")) -> ()
        n269 = global write "Robot Global Data.vi" "y"(0.0 ("y")) -> ()
        n270 = Wait (ms)(milliseconds to wait=u32 0) -> ()  [unwired: 1 out]
      }
      n271 = while {
        tunnel: w261 -> [w292]
        tunnel: [w292] -> w262
        i -> [w287]
        stop <- w286 stop-if-true
        # "Start Shoot."
        n272 = global read "Robot Global Data.vi" "auto shot increase time RED"() -> (w285:i32)
        n273 = Wait (ms)(milliseconds to wait=u32 20) -> ()  [unwired: 1 out]
        n274 = Greater?(x=w287, y=w285) -> (0:w286:bool)
        n275 = global write "Robot Global Data.vi" "Shoot!"(TRUE ("Spinup shooter")) -> ()
        n276 = global write "Robot Global Data.vi" "x"(0.0 ("x")) -> ()
        n277 = global write "Robot Global Data.vi" "z"(0.0 ("z")) -> ()
      }
      n278 = while {
        tunnel: w262 -> [w284]
        tunnel: [w284] -> _
        tunnel: [w282] -> _
        stop <- w282 stop-if-true
        w282 = FALSE
        # "Shoot for remainder of auto."
        n279 = global read "Robot Global Data.vi" "R60P1 shotEnc"() -> (w280:dbl)
        n280 = Wait (ms)(milliseconds to wait=u32 20) -> ()  [unwired: 1 out]
        n281 = global read "Robot Global Data.vi" "FF R60 P1"() -> (w281:dbl)
        n282 = global write "Robot Global Data.vi" "feed forward far"(w281) -> ()
        n283 = global write "Robot Global Data.vi" "shot enc target far"(w280) -> ()
      }
    }
    frame 13 {
      # "Red Auto Doesn't Trigger Hopper"
      # "r60 doesnt trigger"
      # "uses from dashboard:\nshot voltage (feed forward)\nshot encoder target\ninitial y depth\npull forward y depth\ninitial x speed"
      # ".71 FF\n.75 hop"
      # "Red 60 P1"
      n284 = while {
        tunnel: w426 -> [_]
        tunnel: [w546] -> _
        tunnel: [w545] -> w423
        tunnel: w425 -> [w545]
        tunnel: [w544] -> w421
        tunnel: w424 -> [w544]
        stop <- w546 stop-if-true
        # "-21"
        # "Drive Y  until encoder #\nGyro PID for straightness"
        n285 = global read "Robot Global Data.vi" "auto shot increase power RED"() -> (w538:dbl)
        n286 = global read "Robot Global Data.vi" "heading"() -> (w552:dbl)
        n287 = global read "Robot Global Data.vi" "R60P1 shotEnc"() -> (w535:dbl)
        n288 = global read "Robot Global Data.vi" "FF R60 P1"() -> (w534:dbl)
        n289 = global read "Robot Global Data.vi" "encYpos"() -> (w549:dbl)
        n290 = Wait (ms)(milliseconds to wait=u32 20) -> ()  [unwired: 1 out]
        n291 = call-poly <vilib>:"PID.vi"("output range"=cluster{"output high":dbl, "output low":dbl} {"output high"=0.7, "output low"=-0.7}, "PID gains"=T7 {"proportional gain (Kc)"=0.05, "integral time (Ti, min)"=0.007, "derivative time (Td, min)"=0.001}, "process variable"=w552, "setpoint"=0.0) -> ("output"=w550:dbl)  [unwired: 6 in, 1 out]
        n292 = global write "Robot Global Data.vi" "z"(w550) -> ()
        n293 = Less?(x=w549, y=-15.0) -> (x < y?=w546:bool)
        n294 = Multiply(x=w538, y=1000.0) -> (x*y=w536:dbl)
        n295 = Add(x=w538, y=w534) -> (x+y=w539:dbl)
        n296 = global write "Robot Global Data.vi" "Spinup shooter"(TRUE ("Spinup shooter")) -> ()
        n297 = global write "Robot Global Data.vi" "Shot Distance"(TRUE ("Spinup shooter")) -> ()
        n298 = Add(x=w536, y=w535) -> (x+y=w533:dbl)
        n299 = global write "Robot Global Data.vi" "hopper far"(0.75 ("hopper far")) -> ()
        n300 = global write "Robot Global Data.vi" "feed forward far"(w539) -> ()
        n301 = global write "Robot Global Data.vi" "shot enc target far"(w533) -> ()
        n302 = global write "Robot Global Data.vi" "y"(1.0 ("y")) -> ()
      }
      n303 = while {
        tunnel: [w475] -> w422
        tunnel: w423 -> [w475]
        tunnel: w421 -> [w472]
        tunnel: [w472] -> w420
        stop <- TRUE stop-if-true
        # "Empty loop"
        n304 = Wait (ms)(milliseconds to wait=u32 0) -> ()  [unwired: 1 out]
        n305 = global write "Robot Global Data.vi" "y"(0.0 ("y")) -> ()
      }
      n306 = while {
        tunnel: [w532] -> w419
        tunnel: w422 -> [w532]
        tunnel: w420 -> [w531]
        tunnel: [w531] -> w418
        tunnel: [w524] -> _
        stop <- w524 stop-if-true
        # "-.7"
        # "Y to 0\nMove Intake Out of Stow\nArticulate side-wall out\nDrive X at Max until encoder\nGyro PID"
        n307 = global read "Robot Global Data.vi" "no trigger y depth"() -> (w514:dbl)
        n308 = global read "Robot Global Data.vi" "heading"() -> (w528:dbl)
        n309 = global read "Robot Global Data.vi" "encYpos"() -> (w521:dbl)
        n310 = global read "Robot Global Data.vi" "encYpos"() -> (w525:dbl)
        n311 = global read "Robot Global Data.vi" "R60P1 X"() -> (w517:dbl)
        n312 = Add(x=w514, y=1.0) -> (x+y=w516:dbl)
        n313 = call-poly <vilib>:"PID.vi"("output range"=cluster{"output high":dbl, "output low":dbl} {"output high"=0.7, "output low"=-0.7}, "PID gains"=T7 {"proportional gain (Kc)"=0.05, "integral time (Ti, min)"=0.007, "derivative time (Td, min)"=0.001}, "process variable"=w528, "setpoint"=-1.0) -> ("output"=w526:dbl)  [unwired: 6 in, 1 out]
        n314 = Wait (ms)(milliseconds to wait=u32 20) -> ()  [unwired: 1 out]
        n315 = call-poly <vilib>:"PID.vi"("output range"=cluster{"output high":dbl, "output low":dbl} {"output high"=0.5, "output low"=-0.5}, "PID gains"=T7 {"proportional gain (Kc)"=0.03, "integral time (Ti, min)"=0.0, "derivative time (Td, min)"=0.0}, "process variable"=w521, "setpoint"=w514) -> ("output"=w519:dbl)  [unwired: 6 in, 1 out]
        n316 = Less?(x=w525, y=w516) -> (x < y?=w524:bool)
        n317 = global write "Robot Global Data.vi" "z"(w526) -> ()
        n318 = global write "Robot Global Data.vi" "x"(w517) -> ()
        n319 = Negate(x=w519) -> (-x=w518:dbl)
        n320 = global write "Robot Global Data.vi" "y"(w518) -> ()
      }
      n321 = while {
        tunnel: [w499] -> w417
        tunnel: [w498] -> w416
        shift-right: [w510] -> _
        shift-left: _ -> [w509]
        shift-left: _ -> [_]
        shift-left: _ -> [_]
        shift-left: _ -> [_]
        shift-left: _ -> [w505]
        tunnel: w419 -> [w499]
        tunnel: w418 -> [w498]
        i -> [w501]
        stop <- w504 stop-if-true
        # "Stop PID\nLet robot crash into hopper\nand self align to wall.\nStop on time (loop cycles)\nSpin-Up Shooter"
        n322 = global read "Robot Global Data.vi" "R60P1yDepth"() -> (w492:dbl)
        n323 = global read "Robot Global Data.vi" "encYpos"() -> (w496:dbl)
        n324 = Subtract(x=w509, y=w505) -> (x-y=w508:dbl)
        n325 = Absolute Value(x=w508) -> (abs(x)=w507:dbl)
        n326 = Greater?(x=w501, y=6) -> (0:w503:bool)
        n327 = global read "Robot Global Data.vi" "encXpos"() -> (w510:dbl)
        n328 = Wait (ms)(milliseconds to wait=u32 20) -> ()  [unwired: 1 out]
        n329 = Less?(x=w507, y=0.5) -> (x < y?=w502:bool)
        n330 = call-poly <vilib>:"PID.vi"("output range"=cluster{"output high":dbl, "output low":dbl} {"output high"=0.3, "output low"=-0.3}, "PID gains"=T7 {"proportional gain (Kc)"=0.03, "integral time (Ti, min)"=0.0, "derivative time (Td, min)"=0.0}, "process variable"=w496, "setpoint"=w492) -> ("output"=w494:dbl)  [unwired: 6 in, 1 out]
        n331 = Negate(x=w494) -> (-x=w493:dbl)
        n332 = global write "Robot Global Data.vi" "z"(0.0 ("y")) -> ()
        n333 = global write "Robot Global Data.vi" "x"(-1.0 ("x")) -> ()
        n334 = And(x=w502, y=w503) -> (x .and. y?=w504:bool)
        n335 = global write "Robot Global Data.vi" "y"(w493) -> ()
      }
      n336 = while {
        tunnel: [w488] -> w414
        tunnel: w417 -> [w488]
        tunnel: [w487] -> w415
        tunnel: w416 -> [w487]
        i -> [w477]
        stop <- w483 stop-if-true
        # "Let robot pull forward to\ncatch balls.\nStop strafing."
        # "-0.3"
        # "82"
        # "-76"
        n337 = global read "Robot Global Data.vi" "no trigger pullback"() -> (w476:dbl)
        n338 = global read "Robot Global Data.vi" "Vbat"() -> (w479:dbl)
        n339 = global read "Robot Global Data.vi" "encYpos"() -> (w484:dbl)
        n340 = disable-structure shown="Disabled" {
          disable-tunnel: w477 -> [w490 _]
          frame Disabled {
            n341 = Greater?(x=w490, y=10) -> (0:w489:bool)
            n342 = global write "Robot Global Data.vi" "Shoot!"(w489) -> ()
          }
          frame Enabled {
          }
        }
        n343 = Multiply(x=0.19 ("y"), y=12.0) -> (x*y=w481:dbl)
        n344 = Divide(x=w481, y=w479) -> (x/y=w478:dbl)
        n345 = Less?(x=w484, y=w476) -> (x < y?=w483:bool)
        n346 = global write "Robot Global Data.vi" "y"(w478) -> ()
        n347 = global write "Robot Global Data.vi" "x"(0.0 ("x")) -> ()
        n348 = Wait (ms)(milliseconds to wait=u32 20) -> ()  [unwired: 1 out]
      }
      n349 = while {
        tunnel: [w470] -> w413
        tunnel: w414 -> [w470]
        tunnel: w415 -> [w467]
        tunnel: [w467] -> w412
        stop <- TRUE stop-if-true
        # "Stop driving forward"
        n350 = Wait (ms)(milliseconds to wait=u32 20) -> ()  [unwired: 1 out]
        n351 = global write "Robot Global Data.vi" "z"(0.0 ("y")) -> ()
        n352 = global write "Robot Global Data.vi" "x"(0.0 ("y")) -> ()
        n353 = global write "Robot Global Data.vi" "y"(0.0 ("y")) -> ()
      }
      n354 = while {
        tunnel: [w457] -> w411
        tunnel: w413 -> [w457]
        tunnel: [w456] -> w410
        tunnel: w412 -> [w456]
        i -> [w449]
        stop <- w448 stop-if-true
        n355 = disable-structure shown="Disabled" {
          frame Disabled {
            n356 = global read "Robot Global Data.vi" "heading"() -> (w461:dbl)
            n357 = call-poly <vilib>:"PID.vi"("output range"=cluster{"output high":dbl, "output low":dbl} {"output high"=0.7, "output low"=-0.7}, "PID gains"=T7 {"proportional gain (Kc)"=0.05, "integral time (Ti, min)"=0.007, "derivative time (Td, min)"=0.001}, "process variable"=w461, "setpoint"=-4.0) -> ("output"=w459:dbl)  [unwired: 6 in, 1 out]
            n358 = global write "Robot Global Data.vi" "z"(w459) -> ()
          }
          frame Enabled {
          }
        }
        n359 = global read "Robot Global Data.vi" "finished aim?"() -> (w452:bool)
        n360 = Greater?(x=w449, y=50) -> (0:w451:bool)
        n361 = global write "Robot Global Data.vi" "Shoot!"(TRUE ("Spinup shooter")) -> ()
        n362 = global write "Robot Global Data.vi" "autoaim"(TRUE ("autoaim")) -> ()
        n363 = Or(x=w452, y=w451) -> (x .or. y?=w448:bool)
        n364 = global write "Robot Global Data.vi" "y"(0.0 ("y")) -> ()
        n365 = global write "Robot Global Data.vi" "x"(0.0 ("x")) -> ()
        n366 = Wait (ms)(milliseconds to wait=u32 20) -> ()  [unwired: 1 out]
      }
      n367 = while {
        tunnel: [w446] -> w408
        tunnel: w411 -> [w446]
        tunnel: [w445] -> _
        tunnel: w410 -> [w445]
        stop <- TRUE stop-if-true
        # "Pause to let shooter recover from\nrobot movement."
        n368 = global write "Robot Global Data.vi" "autoaim"(FALSE ("autoaim")) -> ()
        n369 = global write "Robot Global Data.vi" "x"(0.0 ("x")) -> ()
        n370 = global write "Robot Global Data.vi" "y"(0.0 ("y")) -> ()
        n371 = Wait (ms)(milliseconds to wait=u32 0) -> ()  [unwired: 1 out]
      }
      n372 = while {
        tunnel: w408 -> [w439]
        tunnel: [w439] -> w409
        i -> [w434]
        stop <- w433 stop-if-true
        # "Start Shoot."
        n373 = global read "Robot Global Data.vi" "auto shot increase time RED"() -> (w432:i32)
        n374 = Wait (ms)(milliseconds to wait=u32 20) -> ()  [unwired: 1 out]
        n375 = Greater?(x=w434, y=w432) -> (0:w433:bool)
        n376 = global write "Robot Global Data.vi" "Shoot!"(TRUE ("Spinup shooter")) -> ()
        n377 = global write "Robot Global Data.vi" "x"(0.0 ("x")) -> ()
        n378 = global write "Robot Global Data.vi" "z"(0.0 ("z")) -> ()
      }
      n379 = while {
        tunnel: w409 -> [w431]
        tunnel: [w431] -> _
        tunnel: [w429] -> _
        stop <- w429 stop-if-true
        w429 = FALSE
        # "Shoot for remainder of auto."
        n380 = global read "Robot Global Data.vi" "R60P1 shotEnc"() -> (w427:dbl)
        n381 = Wait (ms)(milliseconds to wait=u32 20) -> ()  [unwired: 1 out]
        n382 = global read "Robot Global Data.vi" "FF R60 P1"() -> (w428:dbl)
        n383 = global write "Robot Global Data.vi" "feed forward far"(w428) -> ()
        n384 = global write "Robot Global Data.vi" "shot enc target far"(w427) -> ()
      }
    }
    frame 12 {
      # "Move Forward"
      # "Red 60 P1"
      n385 = while {
        tunnel: [w576] -> w556
        tunnel: w558 -> [w576]
        tunnel: [w575] -> w555
        tunnel: w557 -> [w575]
        stop <- w571 stop-if-true
        # "Drive Y  until encoder #\nGyro PID for straightness"
        n386 = global read "Robot Global Data.vi" "heading"() -> (w568:dbl)
        n387 = Wait (ms)(milliseconds to wait=u32 20) -> ()  [unwired: 1 out]
        n388 = global read "Robot Global Data.vi" "encYpos"() -> (w573:dbl)
        n389 = call-poly <vilib>:"PID.vi"("output range"=cluster{"output high":dbl, "output low":dbl} {"output high"=0.7, "output low"=-0.7}, "PID gains"=T7 {"proportional gain (Kc)"=0.06, "integral time (Ti, min)"=0.007, "derivative time (Td, min)"=0.001}, "process variable"=w568, "setpoint"=0.0) -> ("output"=w566:dbl)  [unwired: 6 in, 1 out]
        n390 = Greater?(x=w573, y=100.0) -> (0:w571:bool)
        n391 = global write "Robot Global Data.vi" "y"(-0.8 ("y")) -> ()
        n392 = global write "Robot Global Data.vi" "z"(w566) -> ()
        n393 = global write "Robot Global Data.vi" "x"(0.0 ("x")) -> ()
      }
      n394 = while {
        tunnel: [w563] -> _
        tunnel: w556 -> [w563]
        tunnel: [w562] -> _
        tunnel: w555 -> [w562]
        stop <- FALSE stop-if-true
        w560 = 0.0 ("x")
        # "Drive Y  until encoder #\nGyro PID for straightness"
        n395 = Wait (ms)(milliseconds to wait=u32 20) -> ()  [unwired: 1 out]
        n396 = global write "Robot Global Data.vi" "z"(w560) -> ()
        n397 = global write "Robot Global Data.vi" "y"(w560) -> ()
        n398 = global write "Robot Global Data.vi" "x"(w560) -> ()
      }
    }
    frame 6 {
      # "Red Position 2 (never been run)"
      # "uses from dashboard:\nshot voltage (feed forward)\nshot encoder target\ninitial y depth\npull forward y depth\ninitial x speed"
      # "R60 P2"
      # "Red 60 - P2"
      n399 = while {
        tunnel: w594 -> [_]
        tunnel: [w709] -> _
        tunnel: [w712] -> w588
        tunnel: w593 -> [w712]
        tunnel: [w711] -> w587
        tunnel: w592 -> [w711]
        stop <- w709 stop-if-true
        # "-21"
        # "Drive Y  until encoder #\nGyro PID for straightness"
        n400 = global read "Robot Global Data.vi" "auto shot increase power RED"() -> (w703:dbl)
        n401 = global read "Robot Global Data.vi" "FF R60 P2"() -> (w706:dbl)
        n402 = global read "Robot Global Data.vi" "R60P2 shotEnc"() -> (w700:dbl)
        n403 = global read "Robot Global Data.vi" "encYpos"() -> (w715:dbl)
        n404 = global read "Robot Global Data.vi" "heading"() -> (w718:dbl)
        n405 = Less?(x=w715, y=-10.0) -> (x < y?=w709:bool)
        n406 = Wait (ms)(milliseconds to wait=u32 20) -> ()  [unwired: 1 out]
        n407 = call-poly <vilib>:"PID.vi"("output range"=cluster{"output high":dbl, "output low":dbl} {"output high"=0.7, "output low"=-0.7}, "PID gains"=T7 {"proportional gain (Kc)"=0.05, "integral time (Ti, min)"=0.007, "derivative time (Td, min)"=0.001}, "process variable"=w718, "setpoint"=0.0) -> ("output"=w716:dbl)  [unwired: 6 in, 1 out]
        n408 = global write "Robot Global Data.vi" "Spinup shooter"(TRUE ("Spinup shooter")) -> ()
        n409 = global write "Robot Global Data.vi" "z"(w716) -> ()
        n410 = global write "Robot Global Data.vi" "hopper far"(0.75 ("hopper far")) -> ()
        n411 = global write "Robot Global Data.vi" "y"(1.0 ("y")) -> ()
        n412 = Multiply(x=w703, y=1000.0) -> (x*y=w701:dbl)
        n413 = Add(x=w703, y=w706) -> (x+y=w705:dbl)
        n414 = Add(x=w701, y=w700) -> (x+y=w704:dbl)
        n415 = global write "Robot Global Data.vi" "feed forward far"(w705) -> ()
        n416 = global write "Robot Global Data.vi" "shot enc target far"(w704) -> ()
      }
      n417 = while {
        tunnel: [w653] -> _
        tunnel: [w656] -> w590
        tunnel: w588 -> [w656]
        tunnel: [w655] -> w589
        tunnel: w587 -> [w655]
        stop <- w653 stop-if-true
        w653 = TRUE
        # "Empty Loop"
        n418 = Wait (ms)(milliseconds to wait=u32 0) -> ()  [unwired: 1 out]
      }
      n419 = while {
        tunnel: [w699] -> w581
        tunnel: w590 -> [w699]
        tunnel: w589 -> [w698]
        tunnel: [w698] -> w580
        tunnel: [w689] -> _
        stop <- w689 stop-if-true
        # ".35"
        # "0.03"
        n420 = global read "Robot Global Data.vi" "heading"() -> (w693:dbl)
        n421 = global read "Robot Global Data.vi" "R60P2yDepth"() -> (w679:dbl)
        n422 = Wait (ms)(milliseconds to wait=u32 20) -> ()  [unwired: 1 out]
        n423 = global read "Robot Global Data.vi" "encYpos"() -> (w686:dbl)
        n424 = call-poly <vilib>:"PID.vi"("output range"=cluster{"output high":dbl, "output low":dbl} {"output high"=0.7, "output low"=-0.7}, "PID gains"=T7 {"proportional gain (Kc)"=0.05, "integral time (Ti, min)"=0.007, "derivative time (Td, min)"=0.001}, "process variable"=w693, "setpoint"=0.0) -> ("output"=w691:dbl)  [unwired: 6 in, 1 out]
        n425 = global read "Robot Global Data.vi" "R60P2 X"() -> (w677:dbl)
        n426 = Add(x=w679, y=1.0) -> (x+y=w680:dbl)
        n427 = global read "Robot Global Data.vi" "encYpos"() -> (w690:dbl)
        n428 = global write "Robot Global Data.vi" "Arm Stow"(FALSE ("Arm Stow")) -> ()
        n429 = global write "Robot Global Data.vi" "z"(w691) -> ()
        n430 = global write "Robot Global Data.vi" "Shot Distance"(TRUE ("Spinup shooter")) -> ()
        n431 = global write "Robot Global Data.vi" "Arm 2"(TRUE ("Arm 1")) -> ()
        n432 = global write "Robot Global Data.vi" "Arm 1"(FALSE ("Arm 1")) -> ()
        n433 = call-poly <vilib>:"PID.vi"("output range"=cluster{"output high":dbl, "output low":dbl} {"output high"=0.3, "output low"=-0.3}, "PID gains"=T7 {"proportional gain (Kc)"=0.015, "integral time (Ti, min)"=0.0, "derivative time (Td, min)"=0.0}, "process variable"=w686, "setpoint"=w679) -> ("output"=w685:dbl)  [unwired: 6 in, 1 out]
        n434 = global write "Robot Global Data.vi" "x"(w677) -> ()
        n435 = Less?(x=w690, y=w680) -> (x < y?=w689:bool)
        n436 = Negate(x=w685) -> (-x=w684:dbl)
        n437 = global write "Robot Global Data.vi" "y"(w684) -> ()
      }
      n438 = while {
        tunnel: [w638] -> w585
        tunnel: [w637] -> w584
        shift-right: [w649] -> _
        shift-left: _ -> [w648]
        shift-left: _ -> [_]
        shift-left: _ -> [_]
        shift-left: _ -> [_]
        shift-left: _ -> [w644]
        tunnel: w581 -> [w638]
        tunnel: w580 -> [w637]
        i -> [w640]
        stop <- w643 stop-if-true
        # "Hold Y on PID\nLet robot crash into hopper\nand self align to wall.\nStop on time (loop cycles)"
        n439 = global read "Robot Global Data.vi" "R60P2yDepth"() -> (w631:dbl)
        n440 = global read "Robot Global Data.vi" "encYpos"() -> (w635:dbl)
        n441 = Subtract(x=w648, y=w644) -> (x-y=w647:dbl)
        n442 = Absolute Value(x=w647) -> (abs(x)=w646:dbl)
        n443 = call-poly <vilib>:"PID.vi"("output range"=cluster{"output high":dbl, "output low":dbl} {"output high"=0.3, "output low"=-0.3}, "PID gains"=T7 {"proportional gain (Kc)"=0.015, "integral time (Ti, min)"=0.0, "derivative time (Td, min)"=0.0}, "process variable"=w635, "setpoint"=w631) -> ("output"=w633:dbl)  [unwired: 6 in, 1 out]
        n444 = global read "Robot Global Data.vi" "encXpos"() -> (w649:dbl)
        n445 = Greater?(x=w640, y=6) -> (0:w642:bool)
        n446 = Negate(x=w633) -> (-x=w632:dbl)
        n447 = Less?(x=w646, y=0.5) -> (x < y?=w641:bool)
        n448 = global write "Robot Global Data.vi" "z"(0.0 ("y")) -> ()
        n449 = global write "Robot Global Data.vi" "x"(-1.0 ("x")) -> ()
        n450 = And(x=w641, y=w642) -> (x .and. y?=w643:bool)
        n451 = global write "Robot Global Data.vi" "y"(w632) -> ()
        n452 = Wait (ms)(milliseconds to wait=u32 20) -> ()  [unwired: 1 out]
      }
      n453 = while {
        tunnel: [w619] -> w578
        tunnel: w585 -> [w619]
        tunnel: [w618] -> w583
        tunnel: w584 -> [w618]
        i -> [w608]
        stop <- w614 stop-if-true
        # "Pull forward to catch balls"
        n454 = disable-structure shown="Disabled" {
          disable-tunnel: w608 -> [w622 _]
          frame Disabled {
            n455 = Greater?(x=w622, y=10) -> (0:w620:bool)
            n456 = global write "Robot Global Data.vi" "Shoot!"(w620) -> ()
          }
          frame Enabled {
          }
        }
        n457 = global read "Robot Global Data.vi" "Vbat"() -> (w610:dbl)
        n458 = Wait (ms)(milliseconds to wait=u32 20) -> ()  [unwired: 1 out]
        n459 = Multiply(x=-0.2 ("y"), y=12.0) -> (x*y=w612:dbl)
        n460 = Divide(x=w612, y=w610) -> (x/y=w609:dbl)
        n461 = global read "Robot Global Data.vi" "R60P2 y pullup"() -> (w607:dbl)
        n462 = global write "Robot Global Data.vi" "y"(w609) -> ()
        n463 = global read "Robot Global Data.vi" "encYpos"() -> (w615:dbl)
        n464 = global write "Robot Global Data.vi" "x"(0.0 ("x")) -> ()
        n465 = Greater?(x=w615, y=w607) -> (0:w614:bool)
        "Numeric 2" <- w608
      }
      n466 = while {
        tunnel: [w606] -> w582
        tunnel: w578 -> [w606]
        tunnel: [w605] -> _
        tunnel: w583 -> [w605]
        stop <- TRUE stop-if-true
        # "Stop Robot"
        n467 = Wait (ms)(milliseconds to wait=u32 20) -> ()  [unwired: 1 out]
        n468 = global write "Robot Global Data.vi" "x"(0.0 ("x")) -> ()
        n469 = global write "Robot Global Data.vi" "y"(0.0 ("y")) -> ()
        n470 = global write "Robot Global Data.vi" "z"(0.0 ("y")) -> ()
      }
      n471 = while {
        tunnel: [w665] -> w591
        tunnel: [w667] -> w579
        tunnel: w582 -> [w667]
        i -> [w664]
        stop <- w665 stop-if-true
        # "Auto Aim for max 1 second"
        n472 = global read "Robot Global Data.vi" "finished aim?"() -> (w666:bool)
        n473 = global write "Robot Global Data.vi" "autoaim"(TRUE ("autoaim")) -> ()
        n474 = Greater?(x=w664, y=500) -> (0:w663:bool)
        n475 = Or(x=w666, y=w663) -> (x .or. y?=w665:bool)
        n476 = disable-structure shown="Disabled" {
          frame Disabled {
            n477 = global read "Robot Global Data.vi" "heading"() -> (w674:dbl)
            n478 = call-poly <vilib>:"PID.vi"("output range"=cluster{"output high":dbl, "output low":dbl} {"output high"=0.7, "output low"=-0.7}, "PID gains"=T7 {"proportional gain (Kc)"=0.05, "integral time (Ti, min)"=0.007, "derivative time (Td, min)"=0.001}, "process variable"=w674, "setpoint"=-4.0) -> ("output"=w672:dbl)  [unwired: 6 in, 1 out]
            n479 = global write "Robot Global Data.vi" "z"(w672) -> ()
          }
          frame Enabled {
          }
        }
        n480 = global write "Robot Global Data.vi" "y"(0.0 ("x")) -> ()
        n481 = Wait (ms)(milliseconds to wait=u32 20) -> ()  [unwired: 1 out]
        n482 = global write "Robot Global Data.vi" "x"(0.0 ("x")) -> ()
      }
      n483 = while {
        tunnel: w579 -> [w661]
        tunnel: w591 -> [_]
        tunnel: [w661] -> w586
        stop <- TRUE stop-if-true
        # "Small Wait to allow shooter to \nrecover from movement."
        n484 = global write "Robot Global Data.vi" "x"(0.0 ("x")) -> ()
        n485 = global write "Robot Global Data.vi" "y"(0.0 ("x")) -> ()
        n486 = Wait (ms)(milliseconds to wait=u32 500) -> ()  [unwired: 1 out]
      }
      n487 = while {
        tunnel: w586 -> [w630]
        tunnel: [w630] -> w577
        i -> [w625]
        stop <- w624 stop-if-true
        # "Start Shoot."
        n488 = global read "Robot Global Data.vi" "auto shot increase time RED"() -> (w623:i32)
        n489 = Wait (ms)(milliseconds to wait=u32 20) -> ()  [unwired: 1 out]
        n490 = Greater?(x=w625, y=w623) -> (0:w624:bool)
        n491 = global write "Robot Global Data.vi" "Shoot!"(TRUE ("Spinup shooter")) -> ()
        n492 = global write "Robot Global Data.vi" "x"(0.0 ("x")) -> ()
        n493 = global write "Robot Global Data.vi" "z"(0.0 ("z")) -> ()
      }
      n494 = while {
        tunnel: w577 -> [w599]
        tunnel: [w599] -> _
        tunnel: [w597] -> _
        stop <- w597 stop-if-true
        w597 = FALSE
        # "Shoot for remainder of auto."
        n495 = global read "Robot Global Data.vi" "R60P2 shotEnc"() -> (w595:dbl)
        n496 = Wait (ms)(milliseconds to wait=u32 20) -> ()  [unwired: 1 out]
        n497 = global read "Robot Global Data.vi" "FF R60 P2"() -> (w596:dbl)
        n498 = global write "Robot Global Data.vi" "feed forward far"(w596) -> ()
        n499 = global write "Robot Global Data.vi" "shot enc target far"(w595) -> ()
      }
    }
  }
